vi "PH_USB600x_AnalogReader.constructor.vi"(0 "name":string, 2 "data in":string, 5 "error in(no error)":errorcluster) -> (14 "i ref out":refnum<vi>, 16 "data out":string, 19 "error out":errorcluster)   [LabVIEW 2014, in "PH_USB600x_AnalogReader.lvlib"]
doc: "contructor of the DAQ_E_mIO_Scope class"
uses:
  PH_USB600x_AnalogReader.lvlib
  CS_Core/CSApplicationBaseClasses/DeviceBase/DeviceBase.myEventNames.ctl
  CS_Core/CSSystem/CSSystemLib/CSSystemLib.lvlib
  CS_Core/CSApplicationBaseClasses/DeviceBase/DeviceBase.lvlib
  CS_Core/BaseGUI/BaseGUI.lvlib
  CS_Core/CSObj/CSObj.lvlib
  CS_Core/BaseProcess/BaseProcess.lvlib
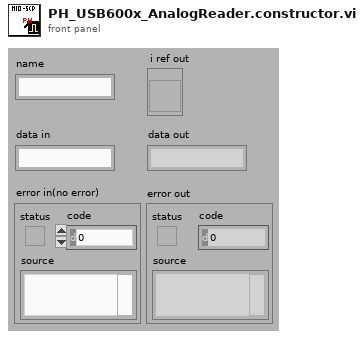
[diagram p1: front panel]
types:
  T1 = enum16{"SetAttribute", "GetAttribute", "CreateAttribute", "DestroyAttribute", "DestroyAllAtributes"}
  T2 = typedef "DeviceBase.lvlib/DeviceBase.myEventNames.ctl" = enum16{"lvmsg://Initialize", "lvmsg://Close", "lvmsg://Configure", "lvmsg://Reset", "lvmsg://IDQuery"}
  T3 = typedef "BaseProcess.lvlib/BaseProcess.i attribute.ctl" = cluster{"EventStatus":string, "EventError":i32, "PresetEvtWatchD":i32, "PresetPdcWatchD":i32, "EventTimeout":i32, "PeriodicInterval":i32, "Interface":string[], "Address":string[], "Special":string[], "PeriodicError":i32, "PeriodicStatus":string, "SuperProc":string, "Descriptors":T4[], "CaseRef":refnum<vi>, "PdcRef":refnum<vi>, "Thread Ref":refnum<vi>, "eventErrorID":i32, "eventStatusID":i32, "periodicErrorID":i32, "periodicStatusID":i32, "pdcCtrID":i32}
  T4 = typedef "BaseProcess.lvlib/BaseProcess.descriptor definition.ctl" = cluster{"selector":string, "descriptor":T5}
  T5 = typedef "BaseProcess.lvlib/BaseProcess.descriptor string definition.ctl" = string
  T6 = typedef "PH_USB600x_AnalogReader.lvlib/PH_USB600x_AnalogReader.i attribute.ctl" = cluster{"GUI Refs":cluster{"Delete":refnum<vi>, "Status":refnum<vi>, "Timeout":refnum<vi>, "Acquire Waveform":refnum<vi>, "Timing":refnum<vi>, "Graph":refnum<vi>, "Prdc Interval":refnum<vi>, "Formula":refnum<vi>}, "Device Settings":cluster{"AIChannel":refnum<k21>, "channelName":string, "Status":T7}, "Timing":T8, "Prdc Interval":dbl, "Lin Scaling":T9, "Data":cluster{"t0":timestamp, dbl}[]}
  T7 = typedef "PH_StatusHandler.lvlib/PH_StatusHandler.Status.ctl" = i16
  T8 = typedef "PH_USB600x_AnalogReader.lvlib/PH_USB600x_AnalogReader.Timing.ctl" = cluster{"Samples per Channel":i32, "Rate":dbl}
  T9 = typedef "PH_USB600x_AnalogReader.lvlib/PH_USB600x_AnalogReader.Lin Scaling.ctl" = cluster{"Slope [Unit/V]":dbl, "Offset [Unit]":dbl, "Y-Unit":string, "Y-Label":string}
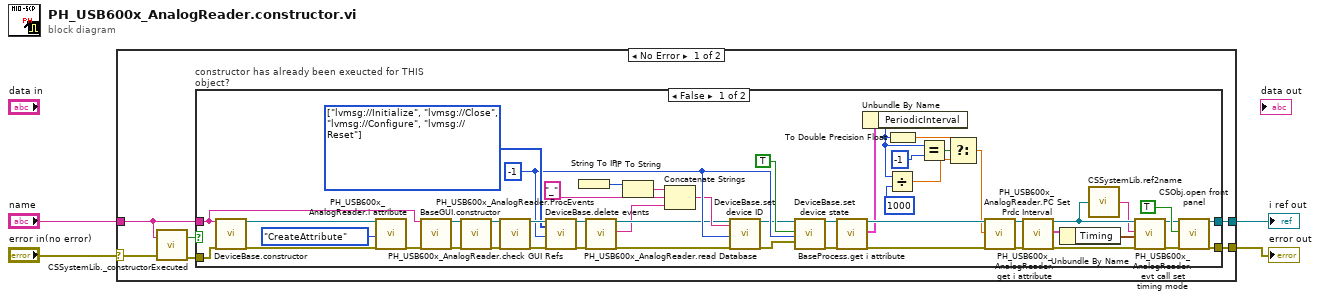
[diagram p0: block diagram]
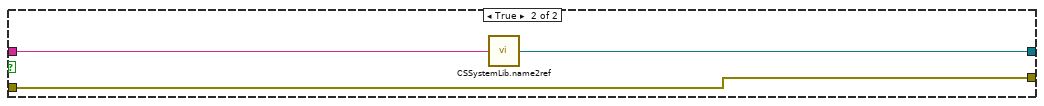
[diagram p2: hidden frame]
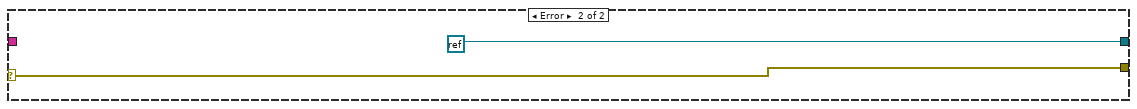
[diagram p3: hidden frame]
diagram:
  n1 = case shown="No Error" "error in(no error)" {
    selector: "error in(no error)" -> [w7 w63]
    tunnel: "name" -> [w6 _]
    tunnel: [w9 refnum<k0> refnum] -> w3
    tunnel: [w8 w63] -> w1
    frame No Error {
      n2 = call "CSSystemLib._constructorExecuted.vi"("name"=w6) -> ("constructor executed?"=w5:bool)  [unwired: 18 in]
      n3 = case "constructor has already been exeucted for THIS object?" shown="False" w5 {
        tunnel: w6 -> [w40 w62]
        tunnel: [w33 w61] -> w9
        tunnel: [w32 w60] -> w8
        tunnel: w7 -> [w56 w60]
        frame False {
          w53 = T2[] [enum."lvmsg://Initialize", enum."lvmsg://Close", enum."lvmsg://Configure", enum."lvmsg://Reset"] items=["lvmsg://Initialize", "lvmsg://Close", "lvmsg://Configure", "lvmsg://Reset", "lvmsg://IDQuery"] ("events")
          w51 = -1 ("ms timeout (10000)")
          n4 = call "DeviceBase.constructor.vi"("name"=w40, "error in (no error)"=w56) -> ("i ref out"=w59:refnum<vi>, "error out"=w58:errorcluster)  [unwired: 15 in, 1 out]
          n5 = call "PH_USB600x_AnalogReader.i attribute.vi"("VI Refnum"=w59, "Action"=T1."CreateAttribute", "error in (no error)"=w58) -> ("error out"=w39:errorcluster)  [unwired: 14 in, 2 out]
          n6 = call "BaseGUI.constructor.vi"("name"=w40, "error in (no error)"=w39) -> ("i ref out"=w38:refnum<vi>, "error out"=w36:errorcluster)  [unwired: 15 in, 1 out]
          n7 = call "PH_USB600x_AnalogReader.check GUI Refs.vi"("i ref in"=w38, "error in (no error)"=w36) -> ("i ref out"=w37:refnum<vi>, "error out"=w35:errorcluster)  [unwired: 15 in, 1 out]
          n8 = call "PH_USB600x_AnalogReader.ProcEvents.vi"("i ref in"=w37, "error in"=w35) -> ("i ref out"=w55:refnum<vi>, "error out"=w54:errorcluster)  [unwired: 16 in]
          n9 = call "DeviceBase.delete events.vi"("i ref in"=w55, "events"=w53, "ms timeout (10000)"=w51, "error in (no error)"=w54) -> ("i ref out"=w44:refnum<vi>, "error out"=w43:errorcluster)  [unwired: 13 in, 1 out]
          n10 = String To IP() -> (0:w50:u32)  [unwired: 1 in]
          n11 = call "PH_USB600x_AnalogReader.read Database.vi"("i ref in"=w44, "error in (no error)"=w43) -> ("i ref out"=w42:refnum<vi>, "Port"=w10:string, "error out"=w41:errorcluster)  [unwired: 15 in]
          n12 = IP To String(2:w50) -> (0:w49:string)  [unwired: 1 in]
          n13 = Concatenate Strings(w49, "_" ("string"), w10) -> (w47:string)
          n14 = call "DeviceBase.set device ID.vi"("i ref in"=w42, "deviceID"=w47, "ms timeout (10000)"=w51, "error in (no error)"=w41) -> ("i ref out"=w46:refnum<vi>, "error out"=w45:errorcluster)  [unwired: 13 in, 1 out]
          n15 = call "DeviceBase.set device state.vi"("i ref in"=w46, "implicit"=TRUE, "ms timeout (10000)"=w51, "device error"=w45) -> ("i ref out"=w20:refnum<vi>, "error out"=w22:errorcluster)  [unwired: 13 in, 1 out]
          n16 = call "BaseProcess.get i attribute.vi"("i ref in"=w20, "error in (no error)"=w22) -> ("i ref out"=w19:refnum<vi>, "i attribute"=w18:T3, "error out"=w21:errorcluster)  [unwired: 15 in]
          n17 = Unbundle By Name(w18) -> ("PeriodicInterval"=w14:i32)
          n18 = Divide(x=w14, y=1000) -> (x/y=w12:dbl)
          n19 = To Double Precision Float(number=w14) -> (double precision float=w13:dbl)
          n20 = Equal?(x=w14, y=-1) -> (x = y?=w16:bool)
          n21 = Select(t=w13, s=w16, f=w12) -> (s? t:f=w11:dbl)
          n22 = call "PH_USB600x_AnalogReader.PC Set Prdc Interval.vi"("i ref in"=w19, "prdc interval [s]"=w11, "error IO"=w21) -> ("i ref out"=w24:refnum<vi>, "error out"=w23:errorcluster)  [unwired: 15 in]
          n23 = call "PH_USB600x_AnalogReader.get i attribute.vi"("i ref in"=w24, "error in (no error)"=w23) -> ("i ref out"=w26:refnum<vi>, "i attribute"=w28:T6, "error out"=w29:errorcluster)  [unwired: 15 in]
          n24 = Unbundle By Name(w28) -> ("Timing"=w27:T8)
          n25 = call "CSSystemLib.ref2name.vi"("obj refnum"=w26) -> ("name"=w25:string)
          n26 = call "PH_USB600x_AnalogReader.evt call set timing mode.vi"("i ref in"=w26, "Instance"=w25, "Timing"=w27, "error in"=w29) -> ("i ref out"=w30:refnum<vi>, "error out"=w31:errorcluster)  [unwired: 14 in]
          n27 = call "CSObj.open front panel.vi"("i ref in"=w30, "frontPanelOpen"=TRUE ("front panel open"), "error in (no error)"=w31) -> ("i ref out"=w33:refnum<vi>, "error out"=w32:errorcluster)  [unwired: 15 in]
        }
        frame True {
          n28 = call "CSSystemLib.name2ref.vi"("name"=w62) -> ("obj refnum"=w61:refnum<vi>)
        }
      }
    }
    frame Error {
    }
  }
  "i ref out" <- w3
  "error out" <- w1
